vi "CORE Insert Assert State Machine.vi"(4 "Cluster":T1, 6 "Eval String":string, 8 "error in (no error)":errorcluster, 11 "Queue in":refnum<queue>) -> (0 "error out":errorcluster)   [LabVIEW 2018]
uses:
  Insert Process Data.ctl
  Save VI Ref Source.ctl
  <vilib>/Utility/traverseref.llb/TRef TravTarget.ctl
  <vilib>/Utility/error.llb/Error Cluster From Error Code.vi
  <vilib>/ErrorRing/Error Ring.xnode
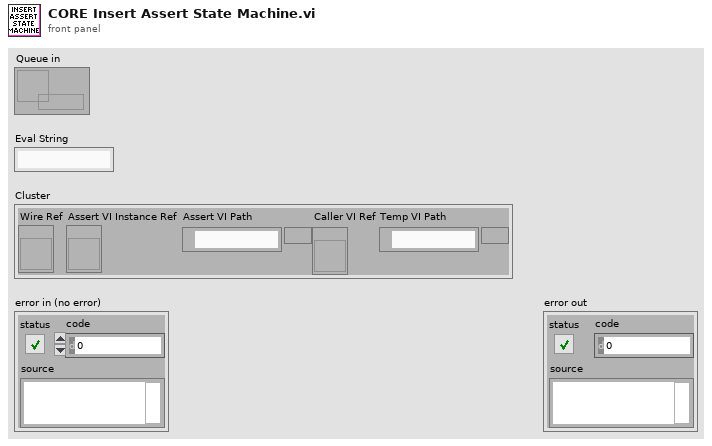
[diagram p1: front panel]
types:
  T1 = typedef "Insert Process Data.ctl" = cluster{"Wire Ref":refnum<vi>, "Assert VI Instance Ref":refnum<vi>, "Assert VI Path":path, "Caller VI Ref":refnum<vi>, "Temp VI Path":path}
  T2 = typedef "Save VI Ref Source.ctl" = enum16{"File Path", "VI Reference"}
  T3 = typedef "TRef TravTarget.ctl" = enum16{"FP", "BD", "Other"}
  T4 = typedef "NewVIObject_LVRelativePositionTypeDef.ctl" = cluster{"Refnum":refnum<vi>, "Relative Direction":T5, "Point32":T6}
  T5 = typedef "NewVIObject_LVRelativeDirectionTypeDef.ctl" = enum32{"Right", "Left", "Top", "Bottom", "Top Right", "Top Left", "Bottom Right", "Bottom Left"}
  T6 = typedef "LVPoint32TypeDef.ctl" = cluster{"Horizontal":i32, "Vertical":i32}
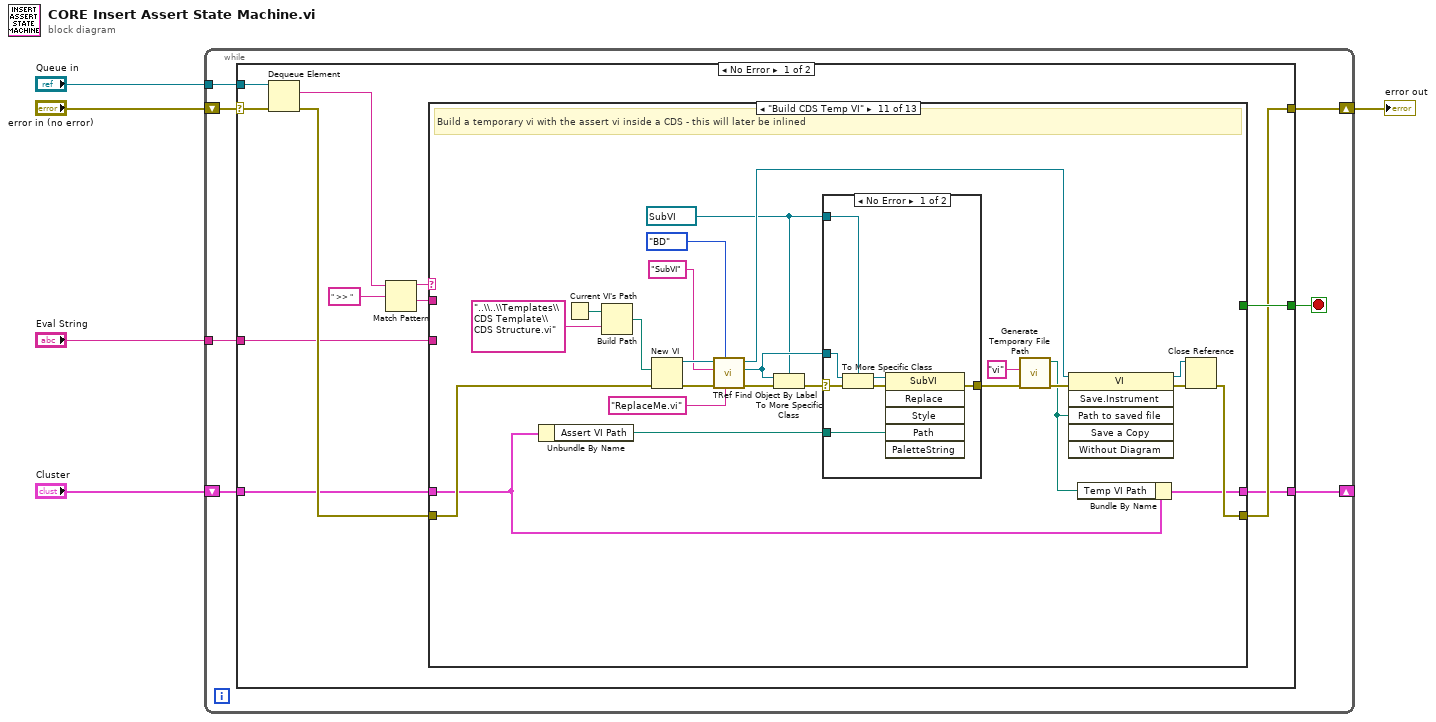
[diagram p0: block diagram]
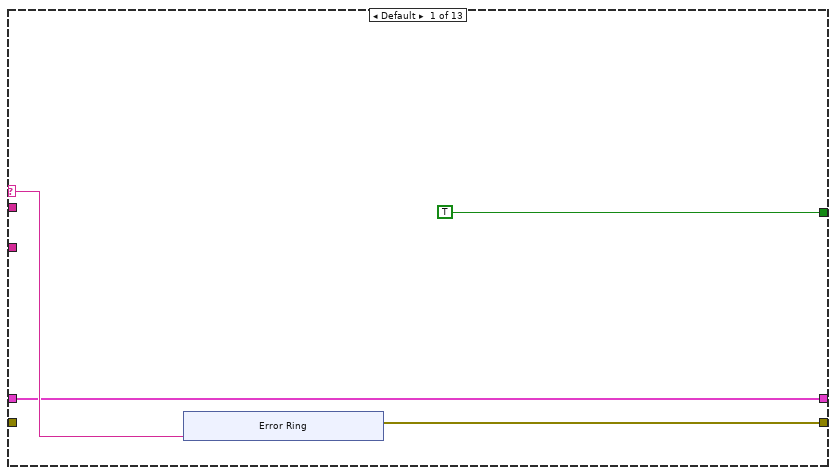
[diagram p2: hidden frame]
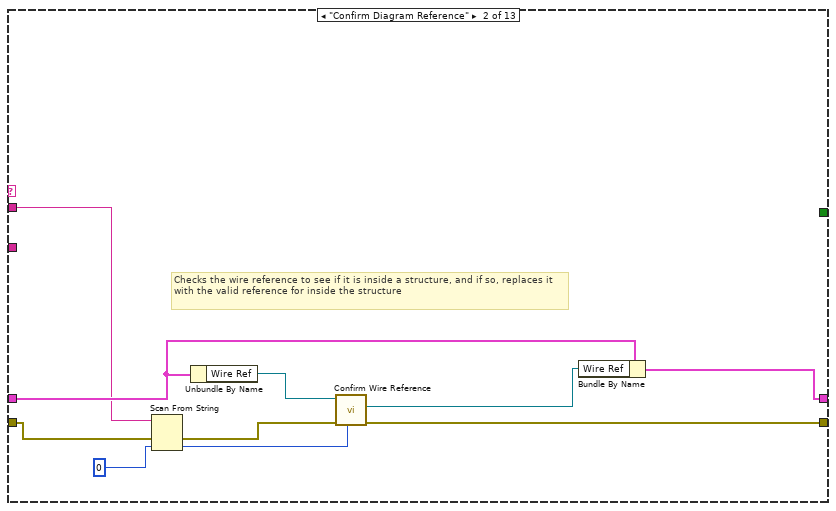
[diagram p3: hidden frame]
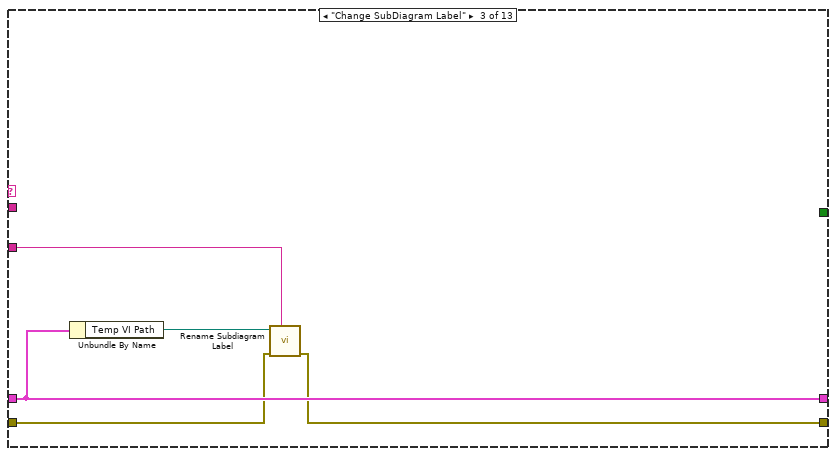
[diagram p4: hidden frame]
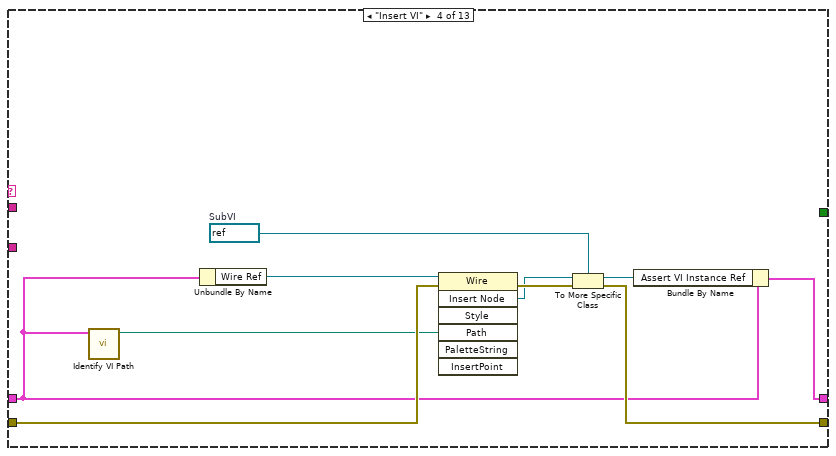
[diagram p5: hidden frame]
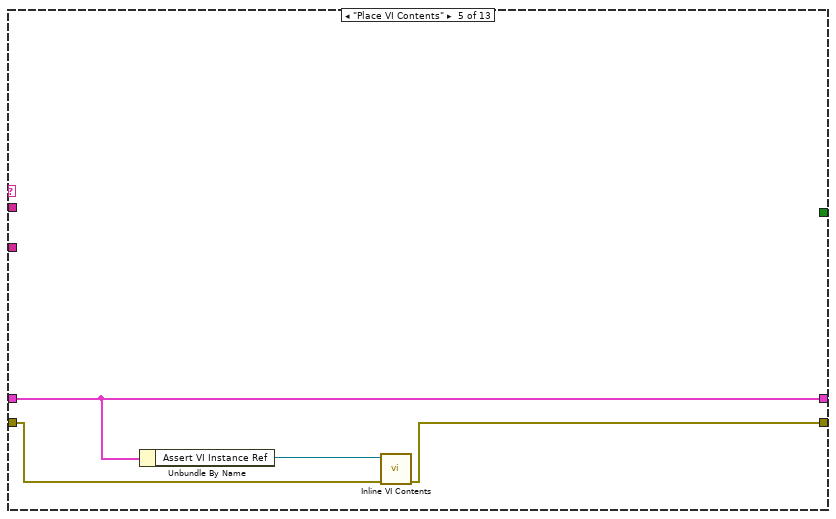
[diagram p6: hidden frame]
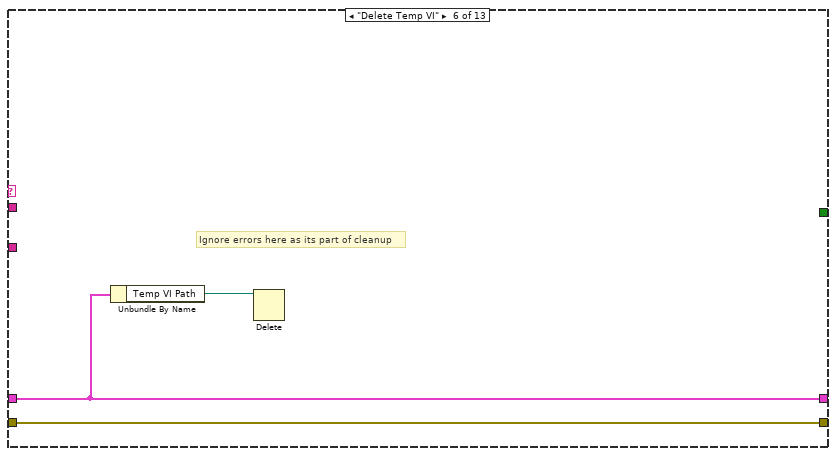
[diagram p7: hidden frame]
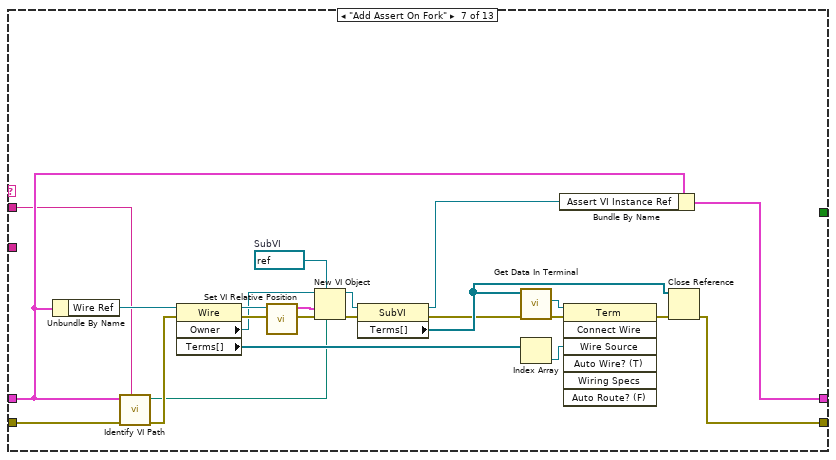
[diagram p8: hidden frame]
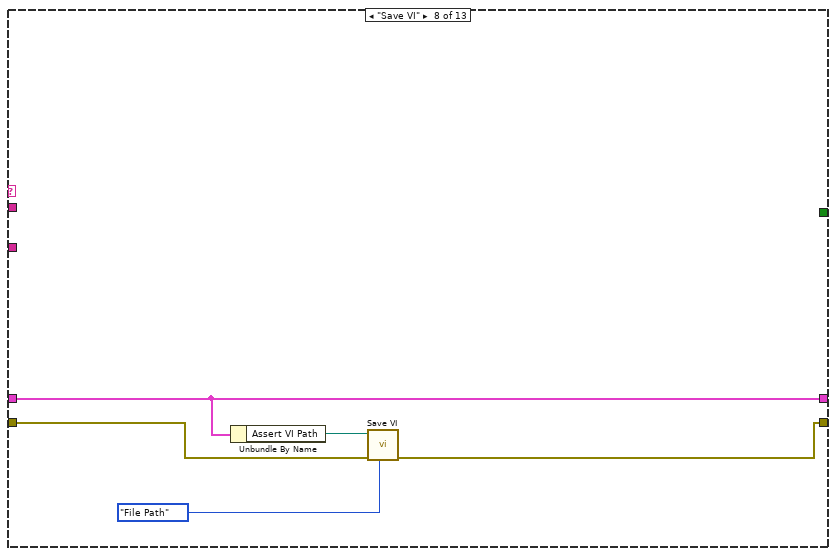
[diagram p9: hidden frame]
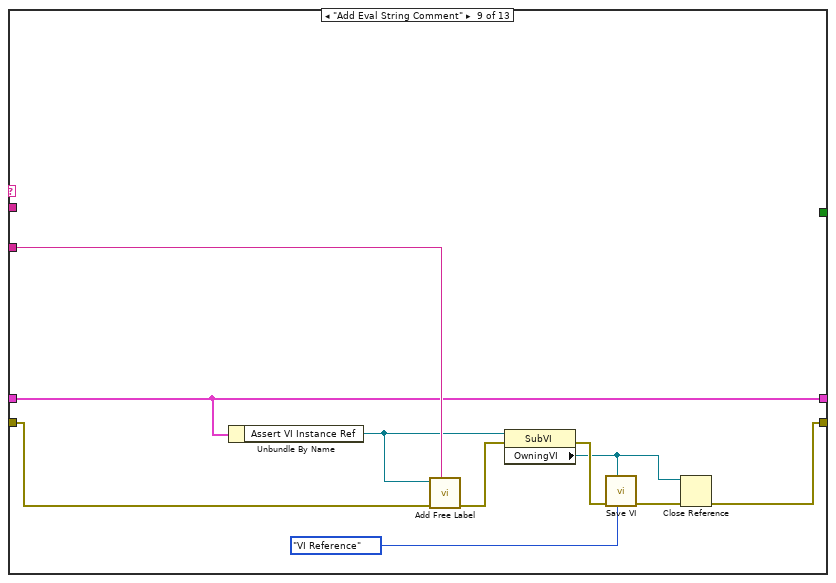
[diagram p10: hidden frame]
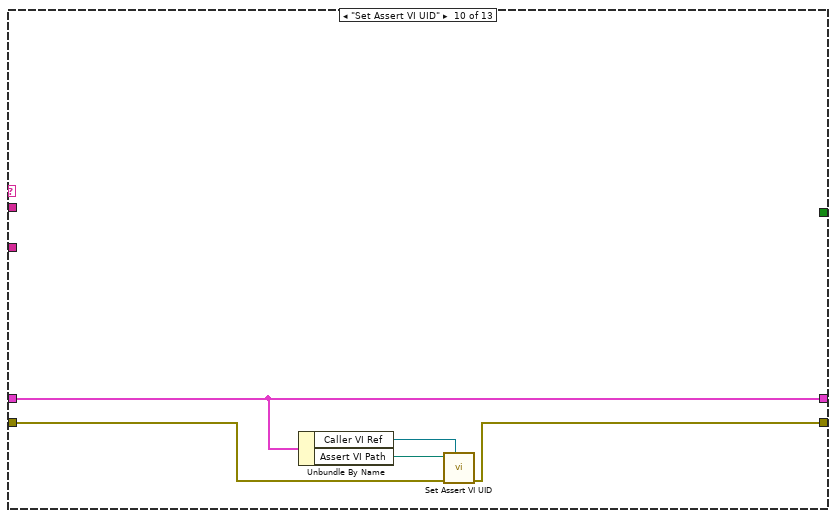
[diagram p11: hidden frame]
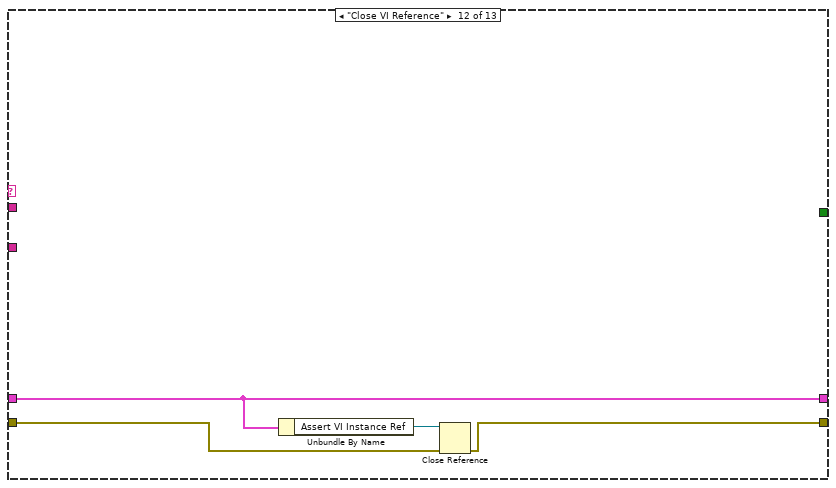
[diagram p13: hidden frame]
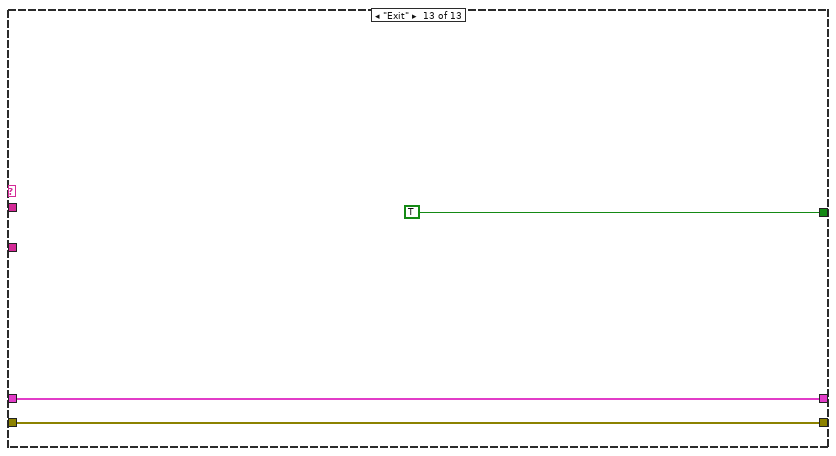
[diagram p14: hidden frame]
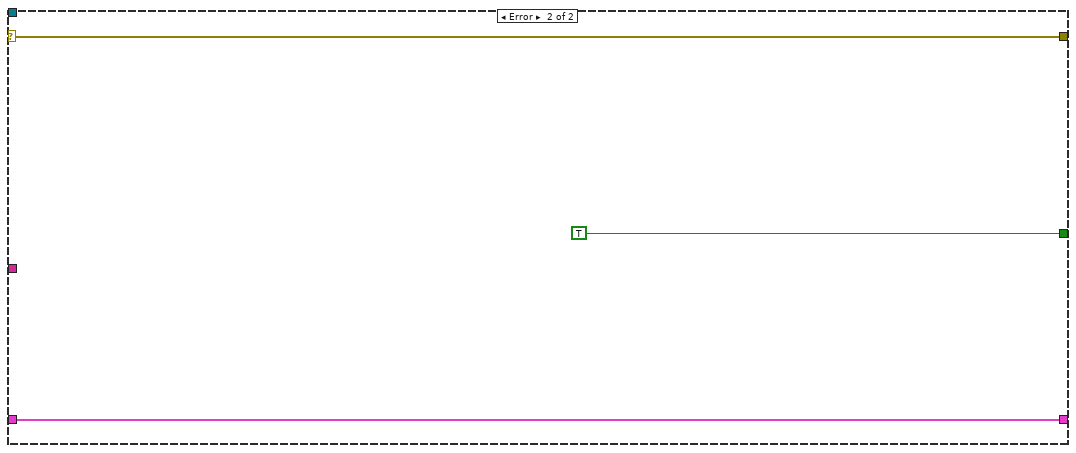
[diagram p15: hidden frame]
diagram:
  n1 = while {
    tunnel: "Queue in" -> [w12]
    shift-right: [w9] -> w5
    shift-left: "error in (no error)" -> [w11]
    shift-right: [w7] -> _
    shift-left: "Cluster" -> [w8]
    tunnel: "Eval String" -> [w6]
    stop <- w10 stop-if-true
    n2 = case shown="No Error" w11 {
      selector: w11 -> [w23 w151]
      tunnel: w12 -> [w24 _]
      tunnel: [w22 TRUE] -> w10
      tunnel: [w20 w151] -> w9
      tunnel: w8 -> [w19 w149]
      tunnel: [w18 w149] -> w7
      tunnel: w6 -> [w17 _]
      frame No Error {
        n3 = Dequeue Element(queue=w24, error in (no error)=w23) -> (element=w16:string, error out=w21:errorcluster)  [unwired: 1 in, 2 out]
        n4 = Match Pattern(string=w16, regular expression=" >> ") -> (before substring=w15:string, after substring=w13:string)  [unwired: 1 in, 2 out]
        n5 = case shown="\"Build CDS Temp VI\"" w15 {
          selector: w15 -> [w27 _ _ _ _ _ _ _ _ _ _ _ _]
          tunnel: [TRUE _ _ _ _ _ _ _ _ _ _ _ TRUE] -> w22
          tunnel: w21 -> [_ w45 w47 w60 w64 w67 w74 w91 w104 w109 w115 w143 w147]
          tunnel: [w26 w44 w46 w58 w61 w67 w73 w90 w95 w105 w112 w142 w147] -> w20
          tunnel: w19 -> [w25 w42 w50 w51 w63 w66 w70 w93 w102 w108 w114 w145 w146]
          tunnel: [w25 w40 w50 w55 w63 w66 w71 w93 w102 w108 w111 w145 w146] -> w18
          tunnel: w17 -> [_ _ w48 _ _ _ _ _ w103 _ _ _ _]
          tunnel: w13 -> [_ w38 _ _ _ _ w68 _ _ _ _ _ _]
          frame Default {
            n6 = xnode "Error Ring"("parameter 0"=w27) -> ("error out"=w26:errorcluster)
          }
          frame "Confirm Diagram Reference" {
            # "Checks the wire reference to see if it is inside a structure, and if so, replaces it with the valid reference for inside the structure"
            n7 = Scan From String(input string=w38, error in=w45, default 1=0) -> (error out=w39:errorcluster, output 1=w36:i32)  [unwired: 2 in, 2 out]
            n8 = Unbundle By Name(w42) -> ("Wire Ref"=w43:refnum<vi>)
            n9 = call "Confirm Wire Reference.vi"("Wire UID"=w36, "error in (no error)"=w39, "Wire in"=w43) -> ("error out"=w44:errorcluster, "Wire Refnum"=w41:refnum<vi>)  [unwired: 7 in]
            n10 = Bundle By Name(cluster=w42, "Wire Ref"=w41) -> (w40:T1)
          }
          frame "Change SubDiagram Label" {
            n11 = Unbundle By Name(w50) -> ("Temp VI Path"=w49:path)
            n12 = call "Rename Subdiagram Label.vi"("Evaluation String"=w48, "error in (no error)"=w47, "VI Path"=w49) -> ("error out"=w46:errorcluster)  [unwired: 8 in]
          }
          frame "Insert VI" {
            w57 = refnum<vi> refnum  # SubVI
            n13 = call "Identify VI Path.vi"("State Data"=w51) -> ("VI Path"=w53:path)  [unwired: 10 in]
            n14 = Unbundle By Name(w51) -> ("Wire Ref"=w52:refnum<vi>)
            n15 = invoke class="Wire" method="Insert Node"(reference=w52, error in=w60, "Path"=w53) -> (error out=w59:errorcluster, "Insert Node"=w54:refnum<vi>)  [unwired: 4 in, 5 out]
            n16 = To More Specific Class(target class=w57, reference=w54, error in=w59) -> (specific class reference=w56:refnum<vi>, error out=w58:errorcluster)
            n17 = Bundle By Name(cluster=w51, "Assert VI Instance Ref"=w56) -> (w55:T1)
          }
          frame "Place VI Contents" {
            n18 = Unbundle By Name(w63) -> ("Assert VI Instance Ref"=w62:refnum<vi>)
            n19 = call "Inline VI Contents.vi"("error in (no error)"=w64, "SubVI in"=w62) -> ("error out"=w61:errorcluster)  [unwired: 9 in]
          }
          frame "Delete Temp VI" {
            # "Ignore errors here as its part of cleanup"
            n20 = Unbundle By Name(w66) -> ("Temp VI Path"=w65:path)
            n21 = Delete(path (use dialog)=w65) -> ()  [unwired: 4 in, 3 out]
          }
          frame "Add Assert On Fork" {
            w89 = refnum<vi> refnum  # SubVI
            n22 = Unbundle By Name(w70) -> ("Wire Ref"=w75:refnum<vi>)
            n23 = call "Identify VI Path.vi"("ID"=w68, "State Data"=w70) -> ("VI Path"=w69:path)  [unwired: 9 in]
            n24 = property class="Wire"(reference=w75, error in=w74) -> (reference out=w80:refnum<vi>, error out=w79:errorcluster, "Owner"=w76:refnum<vi>, "Terms[]"=w77:refnum<vi>[])
            n25 = call "Set VI Relative Position.vi"("Wire in"=w80) -> ("Relative Position"=w88:T4)  [unwired: 10 in]
            n26 = New VI Object(vi object class=w89, owner refnum=w76, position/next to=w88, 6:w69, 8:w79) -> (object refnum=w85:refnum<vi>, 0:w87:errorcluster)  [unwired: 3 in]
            n27 = property class="SubVI"(reference=w85, error in=w87) -> (reference out=w72:refnum<vi>, error out=w82:errorcluster, "Terms[]"=w83:refnum<vi>[])
            n28 = call "Get Data In Terminal.vi"("error in (no error)"=w82, "Terms[]"=w83) -> ("error out"=w84:errorcluster, "Terminal out"=w78:refnum<vi>)  [unwired: 8 in]
            n29 = Index Array(array=w77) -> (element=w81:refnum<vi>)  [unwired: 1 in]
            n30 = Bundle By Name(cluster=w70, "Assert VI Instance Ref"=w72) -> (w71:T1)
            n31 = invoke class="Term" method="Connect Wire"(reference=w78, error in=w84, "Wire Source"=w81) -> (error out=w86:errorcluster)  [unwired: 4 in, 6 out]
            n32 = Close Reference(reference=w83, error in (no error)=w86) -> (error out=w73:errorcluster)
          }
          frame "Save VI" {
            n33 = Unbundle By Name(w93) -> ("Assert VI Path"=w92:path)
            n34 = call "Save VI.vi"("Reference Source"=Save_VI_Ref_Source."File Path", "error in (no error)"=w91, "Assert VI Path"=w92) -> ("error out"=w90:errorcluster)  [unwired: 8 in]
          }
          frame "Add Eval String Comment" {
            n35 = Unbundle By Name(w102) -> ("Assert VI Instance Ref"=w96:refnum<vi>)
            n36 = call "Add Free Label.vi"("Evaluation String"=w103, "error in (no error)"=w104, "Assert VI Refnum"=w96) -> ("error out"=w97:errorcluster)  [unwired: 8 in]
            n37 = property class="SubVI"(reference=w96, error in=w97) -> (error out=w99:errorcluster, "OwningVI"=w98:refnum<vi>)  [unwired: 1 out]
            n38 = call "Save VI.vi"("Reference Source"=Save_VI_Ref_Source."VI Reference", "VI Refnum"=w98, "error in (no error)"=w99) -> ("error out"=w100:errorcluster)  [unwired: 8 in]
            n39 = Close Reference(reference=w98, error in (no error)=w100) -> (error out=w95:errorcluster)
          }
          frame "Set Assert VI UID" {
            n40 = Unbundle By Name(w108) -> ("Caller VI Ref"=w106:refnum<vi>, "Assert VI Path"=w107:path)
            n41 = call "Set Assert VI UID.vi"("Caller VI Ref"=w106, "error in (no error)"=w109, "Assert VI Path"=w107) -> ("error out"=w105:errorcluster)  [unwired: 8 in]
          }
          frame "Build CDS Temp VI" {
            w117 = refnum<vi> refnum ("Found Obj Ref")
            # "Build a temporary vi with the assert vi inside a CDS - this will later be inlined"
            n42 = Unbundle By Name(w114) -> ("Assert VI Path"=w113:path)
            n43 = Current VI's Path() -> (path=w122:path)
            n44 = Build Path(base path=w122, name or relative path="..\\..\\Templates\\CDS Template\\CDS Structure.vi") -> (appended path=w123:path)
            n45 = New VI(8:w115, 10:w123) -> (0:w125:errorcluster, 3:w124:refnum<vi>)  [unwired: 5 in]
            n46 = call <vilib>:"TRef Find Object By Label.vi"("Label"="ReplaceMe.vi", "Traverse Target"=TRef_TravTarget."BD", "error in (no error)"=w125, "Class Name"="SubVI", "VI Ref"=w124) -> ("error out"=w126:errorcluster, "Found Obj Ref"=w128:refnum<vi>, "dup VI Ref"=w131:refnum<vi>)  [unwired: 3 in, 1 out]
            n47 = To More Specific Class(target class=w117, reference=w128, error in=w126) -> (error out=w127:errorcluster)  [unwired: 1 out]
            n48 = case shown="No Error" w127 {
              selector: w127 -> [w138 w141]
              tunnel: w117 -> [w140 _]
              tunnel: w128 -> [w139 _]
              tunnel: [w134 w141] -> w129
              tunnel: w113 -> [w135 _]
              frame No Error {
                n49 = To More Specific Class(target class=w140, reference=w139, error in=w138) -> (specific class reference=w137:refnum<vi>, error out=w136:errorcluster)
                n50 = invoke class="SubVI" method="Replace"(reference=w137, error in=w136, "Path"=w135) -> (error out=w134:errorcluster)  [unwired: 3 in, 5 out]
              }
              frame Error {
                # "Should never happen as the path to the template vi is hard coded"
              }
            }
            n51 = call <vilib>:"Generate Temporary File Path.vi"("error in (no error)"=w129, "Temporary File Extension (tmp)"="vi") -> ("error out"=w130:errorcluster, "Unique Temporary File Path"=w110:path)  [unwired: 8 in]
            n52 = invoke class="VI" method="Save.Instrument"(reference=w131, error in=w130, "Path to saved file"=w110) -> (reference out=w132:refnum<vi>, error out=w133:errorcluster)  [unwired: 3 in, 4 out]
            n53 = Bundle By Name(cluster=w114, "Temp VI Path"=w110) -> (w111:T1)
            n54 = Close Reference(reference=w132, error in (no error)=w133) -> (error out=w112:errorcluster)
          }
          frame "Close VI Reference" {
            n55 = Unbundle By Name(w145) -> ("Assert VI Instance Ref"=w144:refnum<vi>)
            n56 = Close Reference(reference=w144, error in (no error)=w143) -> (error out=w142:errorcluster)
          }
          frame "Exit" {
          }
        }
      }
      frame Error {
      }
    }
  }
  "error out" <- w5
